vi "SP Complex Inverse Matrix.vi"(3 "Input Matrix":T1) -> (0 "error":i32, 1 "Inverse Matrix":T1)   [LabVIEW 2011]
doc: "Finds <B>Inverse Matrix</B>, if it exists, of <B>Input Matrix</B>. The data type you wire to the <B>Input Matrix</B> input determines the polymorphic instance to use."
uses:
  TypeDefs/SP Complex Matrix.ctl
panel:
  # "Complex Inverse Matrix"
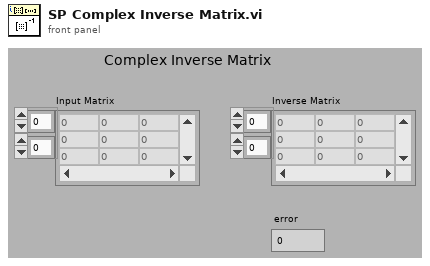
[diagram p1: front panel]
types:
  T1 = typedef "SP Complex Matrix.ctl" = cdb[][]
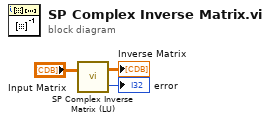
[diagram p0: block diagram]
diagram:
  n1 = call "SP Complex Inverse Matrix (LU).vi"("A"="Input Matrix") -> ("error"=→"error":i32, "Inverse Matrix"=→"Inverse Matrix":T1)  [unwired: 1 out]
